vi "Global.vi"() -> ()   [LabVIEW 2019, in "XCP_DaqDtoId.lvlib" / "DAQList.lvclass"]
uses:
  DAQList.lvclass
panel:
  in  "Meas Split Tag Second":string="__S2_"
  in  "Meas Split Tag First":string="__S1_"
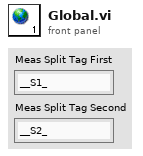
[diagram p1: front panel]
diagram:
